vi "Write to Markdown File.vi"() -> ()   [LabVIEW 2017]
panel:
  in  "Image Name Cluster":T1
  in  "Header Size 2":T2(ring)
  in  "Unformatted Sub-Header Input":string
  in  "Unformatted Header Cluster":T3
  in  "Unformatted Numeric Array":dbl[][](array[numeric])
  in  "Unformatted Paragraph Input":string
  out "output file refnum":refnum<file>
  out "Error Out":errorcluster
  in  "Error In":errorcluster
  in  "Header Size":T2(ring)
  in  "Unformatted Header Input":string
  # "Image Details Input"
  # "Header Input"
  # "Sub-Header Input"
  # "Output"
  # "Paragraph Input"
  # "Table Input"
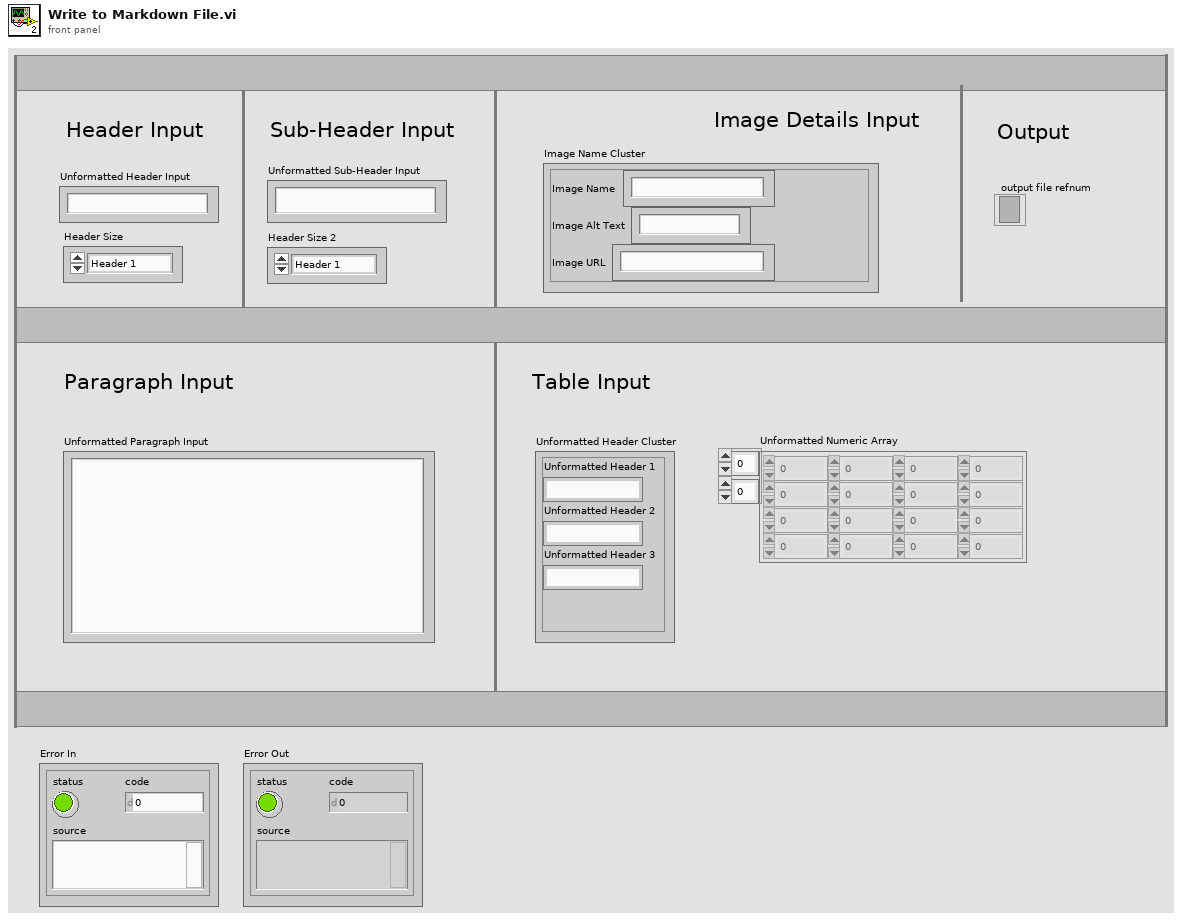
[diagram p1: front panel]
types:
  T1 = cluster{"Image Name":string, "Image Alt Text":string, "Image URL":string}
  T2 = enum16{"Header 1", "Header 2", "Header 3", "Header 4", "Header 5", "Header 6"}
  T3 = cluster{"Unformatted Header 1":string, "Unformatted Header 2":string, "Unformatted Header 3":string}
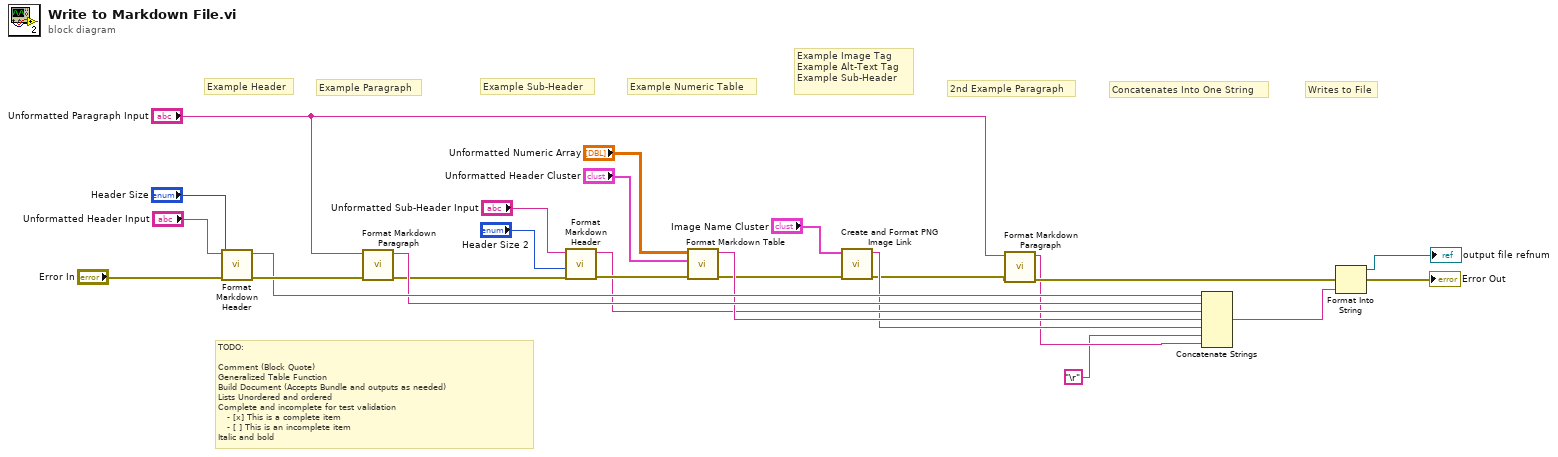
[diagram p0: block diagram]
diagram:
  # "2nd Example Paragraph"
  # "Example Image Tag \nExample Alt-Text Tag \nExample Sub-Header"
  # "TODO:\n\nComment (Block Quote)\nGeneralized Table Function\nBuild Document (Accepts Bundle and outputs as needed)\nLists Unordered and ordered\nComplete and incomplete for test validation\n   - [x] This is a complete item\n   - [ ] This is an incomplete item\nItalic and bold"
  # "Example Sub-Header"
  # "Writes to File"
  # "Concatenates Into One String"
  # "Example Numeric Table"
  # "Example Paragraph"
  # "Example Header"
  n1 = call "Format Markdown Header.vi"("Error In"="Error In", "Header Size"="Header Size", "Unformatted Heading Input"="Unformatted Header Input") -> ("Error Out"=w20:errorcluster, "Formatted Header Output"=w19:string)  [unwired: 7 in]
  n2 = call "Format Markdown Paragraph.vi"("Error In"=w20, "Unformatted Paragraph Input"="Unformatted Paragraph Input") -> ("Error Out"=w14:errorcluster, "Formatted Sentence Output"=w18:string)  [unwired: 8 in]
  n3 = call "Format Markdown Header.vi"("Error In"=w14, "Header Size"="Header Size 2", "Unformatted Heading Input"="Unformatted Sub-Header Input") -> ("Error Out"=w13:errorcluster, "Formatted Header Output"=w9:string)  [unwired: 7 in]
  n4 = call "Format Markdown Table.vi"("Error In"=w13, "Unformatted Header Cluster"="Unformatted Header Cluster", "Unformatted Numeric Array"="Unformatted Numeric Array") -> ("Error Out"=w8:errorcluster, "Formatted Array to Markdown Table"=w10:string)  [unwired: 7 in]
  n5 = call "Create and Format PNG Image Link.vi"("Error In"=w8, "Image Name Cluster"="Image Name Cluster") -> ("Error Out"=w5:errorcluster, "Image Link"=w6:string)  [unwired: 8 in]
  n6 = call "Format Markdown Paragraph.vi"("Error In"=w5, "Unformatted Paragraph Input"="Unformatted Paragraph Input") -> ("Error Out"=w3:errorcluster, "Formatted Sentence Output"=w2:string)  [unwired: 8 in]
  n7 = Concatenate Strings(w19, w18, w9, w10, w6, "\r", w2) -> (w17:string)
  n8 = Format Into String(error in=w3, w17) -> (resulting string=→"output file refnum":refnum<file>, error out=→"Error Out":errorcluster)  [unwired: 2 in]
